vi "SoftwareTimedVoltAcq.vi"() -> ()   [LabVIEW 2014]
uses:
  <vilib>/DAQmx/create/channels.llb/DAQmx Create Channel (AI-Voltage-Basic).vi
  <vilib>/DAQmx/read.llb/DAQmx Read (Analog DBL 1Chan 1Samp).vi
panel:
  in  "CJC Temperature":dbl
  in  "Sample Rate":dbl
  in  "stop":bool
  in  "physical channels":tag
  out "Voltage":dbl(graph)
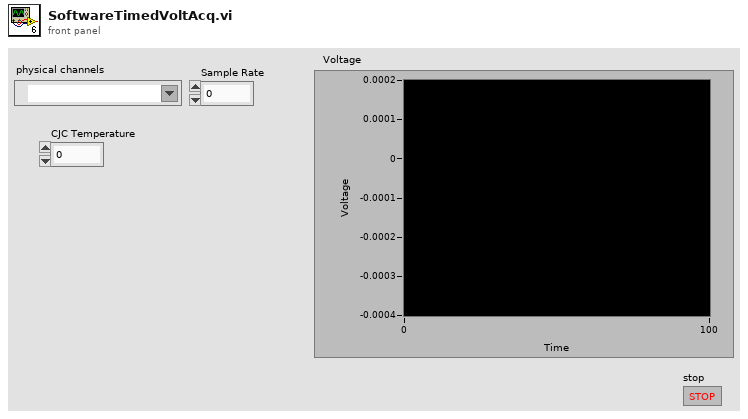
[diagram p1: front panel]
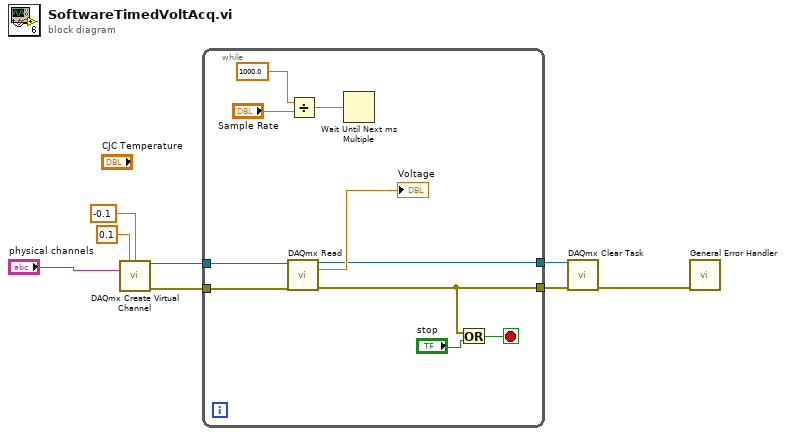
[diagram p0: block diagram]
diagram:
  n1 = call-poly <vilib>:"DAQmx Create Virtual Channel.vi"("maximum value"=0.1, "minimum value"=-0.1, "physical channels"="physical channels") -> ("task out"=w7:refnum<k21>, "error out"=w6:errorcluster)  [unwired: 11 in]
  n2 = while {
    tunnel: w7 -> [w18]
    tunnel: w6 -> [w17]
    tunnel: [w12] -> w3
    tunnel: [w9] -> w2
    stop <- w10 stop-if-true
    n3 = call-poly <vilib>:"DAQmx Read.vi"("task/channels in"=w18, "error in"=w17) -> ("task out"=w12:refnum<k21>, "data"=→"Voltage":dbl, "error out"=w9:errorcluster)  [unwired: 11 in]
    n4 = Divide(x=1000.0, y="Sample Rate") -> (x/y=w13:dbl)
    n5 = Wait Until Next ms Multiple(millisecond multiple=w13) -> ()  [unwired: 1 out]
    n6 = Or(x=w9, y="stop") -> (x .or. y?=w10:bool)
  }
  n7 = call <vilib>:"DAQmx Clear Task.vi"("task in"=w3, "error in"=w2) -> ("error out"=w1:errorcluster)  [unwired: 13 in]
  n8 = call <vilib>:"General Error Handler.vi"("error in (no error)"=w1) -> ()  [unwired: 10 in, 5 out]
